vi "Colour detection subVI.vi"(2 "error in":errorcluster, 3 "Enum":T1(ring), 4 "Image In":T2) -> (0 "error out":errorcluster, 1 "Image overlay":T2(plugin-control))   [LabVIEW 2018]
uses:
  <vilib>/vision/Image Controls.llb/IMAQ Image.ctl
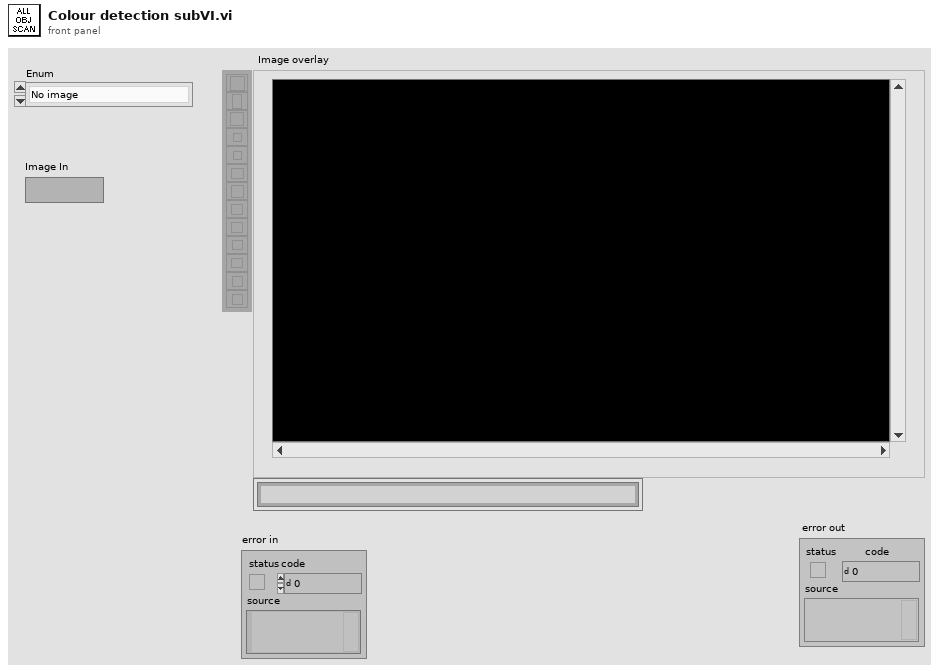
[diagram p1: front panel]
types:
  T1 = enum16{"No image", "Hair gel detection", "Pipe detection", "Ball detection", "Soap detection"}
  T2 = typedef "IMAQ Image.ctl" = refnum<image>
  T3 = cluster{"Desired Font (Application)":enum16{"User-specified Font", "Application Font", "System Font", "Dialog Font"}, "[User-specified Font]":cluster{"Font Name":string, "Size":i16, "Strikeout?":bool, "Italic?":bool, "Underline?":bool, "Outline?":bool, "Shadow?":bool, "Bold?":bool, "Rotation Angle":dbl}, "Horizontal Alignment":i16, "Vertical Alignment":i16}
  T4 = cluster{"Position":cluster{"x":sgl, "y":sgl}, "Angle":sgl, "Scale":sgl, "Score":sgl, "Bounding Box":cluster{"x":sgl, "y":sgl}[]}[]
  T5 = cluster{"Matches (Detect red)[0]":cluster{"Position":cluster{"x":sgl, "y":sgl}, "Angle":sgl, "Scale":sgl, "Score":sgl, "Bounding Box":cluster{"x":sgl, "y":sgl}[]}, "Matches (Detect red)[1]":cluster{"Position":cluster{"x":sgl, "y":sgl}, "Angle":sgl, "Scale":sgl, "Score":sgl, "Bounding Box":cluster{"x":sgl, "y":sgl}[]}, "Matches (Detect red)[2]":cluster{"Position":cluster{"x":sgl, "y":sgl}, "Angle":sgl, "Scale":sgl, "Score":sgl, "Bounding Box":cluster{"x":sgl, "y":sgl}[]}, "Matches (Detect red)[3]":cluster{"Position":cluster{"x":sgl, "y":sgl}, "Angle":sgl, "Scale":sgl, "Score":sgl, "Bounding Box":cluster{"x":sgl, "y":sgl}[]}, "Matches (Detect red)[4]":cluster{"Position":cluster{"x":sgl, "y":sgl}, "Angle":sgl, "Scale":sgl, "Score":sgl, "Bounding Box":cluster{"x":sgl, "y":sgl}[]}, "Matches (Detect red)[5]":cluster{"Position":cluster{"x":sgl, "y":sgl}, "Angle":sgl, "Scale":sgl, "Score":sgl, "Bounding Box":cluster{"x":sgl, "y":sgl}[]}, "Matches (Detect red)[6]":cluster{"Position":cluster{"x":sgl, "y":sgl}, "Angle":sgl, "Scale":sgl, "Score":sgl, "Bounding Box":cluster{"x":sgl, "y":sgl}[]}, "Matches (Detect red)[7]":cluster{"Position":cluster{"x":sgl, "y":sgl}, "Angle":sgl, "Scale":sgl, "Score":sgl, "Bounding Box":cluster{"x":sgl, "y":sgl}[]}, "Matches (Detect red)[8]":cluster{"Position":cluster{"x":sgl, "y":sgl}, "Angle":sgl, "Scale":sgl, "Score":sgl, "Bounding Box":cluster{"x":sgl, "y":sgl}[]}}
  T6 = cluster{"Bounding Box[0]":cluster{"x":sgl, "y":sgl}, "Bounding Box[1]":cluster{"x":sgl, "y":sgl}, "Bounding Box[2]":cluster{"x":sgl, "y":sgl}, "Bounding Box[3]":cluster{"x":sgl, "y":sgl}, "Bounding Box[4]":cluster{"x":sgl, "y":sgl}, "Bounding Box[5]":cluster{"x":sgl, "y":sgl}, "Bounding Box[6]":cluster{"x":sgl, "y":sgl}, "Bounding Box[7]":cluster{"x":sgl, "y":sgl}, "Bounding Box[8]":cluster{"x":sgl, "y":sgl}}
  T7 = cluster{"Global Rectangle":cluster{"x1Left":i32, "y1Top":i32, "x2Right":i32, "y2Bottom":i32}, "Centroid":cluster{"x":sgl, "y":sgl}, "Object Size":u32, "Score":dbl}[]
  T8 = cluster{"Shape Report (Shape Matching 1)[0]":cluster{"Global Rectangle":cluster{"x1Left":i32, "y1Top":i32, "x2Right":i32, "y2Bottom":i32}, "Centroid":cluster{"x":sgl, "y":sgl}, "Object Size":u32, "Score":dbl}, "Shape Report (Shape Matching 1)[1]":cluster{"Global Rectangle":cluster{"x1Left":i32, "y1Top":i32, "x2Right":i32, "y2Bottom":i32}, "Centroid":cluster{"x":sgl, "y":sgl}, "Object Size":u32, "Score":dbl}, "Shape Report (Shape Matching 1)[2]":cluster{"Global Rectangle":cluster{"x1Left":i32, "y1Top":i32, "x2Right":i32, "y2Bottom":i32}, "Centroid":cluster{"x":sgl, "y":sgl}, "Object Size":u32, "Score":dbl}, "Shape Report (Shape Matching 1)[3]":cluster{"Global Rectangle":cluster{"x1Left":i32, "y1Top":i32, "x2Right":i32, "y2Bottom":i32}, "Centroid":cluster{"x":sgl, "y":sgl}, "Object Size":u32, "Score":dbl}, "Shape Report (Shape Matching 1)[4]":cluster{"Global Rectangle":cluster{"x1Left":i32, "y1Top":i32, "x2Right":i32, "y2Bottom":i32}, "Centroid":cluster{"x":sgl, "y":sgl}, "Object Size":u32, "Score":dbl}, "Shape Report (Shape Matching 1)[5]":cluster{"Global Rectangle":cluster{"x1Left":i32, "y1Top":i32, "x2Right":i32, "y2Bottom":i32}, "Centroid":cluster{"x":sgl, "y":sgl}, "Object Size":u32, "Score":dbl}, "Shape Report (Shape Matching 1)[6]":cluster{"Global Rectangle":cluster{"x1Left":i32, "y1Top":i32, "x2Right":i32, "y2Bottom":i32}, "Centroid":cluster{"x":sgl, "y":sgl}, "Object Size":u32, "Score":dbl}, "Shape Report (Shape Matching 1)[7]":cluster{"Global Rectangle":cluster{"x1Left":i32, "y1Top":i32, "x2Right":i32, "y2Bottom":i32}, "Centroid":cluster{"x":sgl, "y":sgl}, "Object Size":u32, "Score":dbl}, "Shape Report (Shape Matching 1)[8]":cluster{"Global Rectangle":cluster{"x1Left":i32, "y1Top":i32, "x2Right":i32, "y2Bottom":i32}, "Centroid":cluster{"x":sgl, "y":sgl}, "Object Size":u32, "Score":dbl}}
  T9 = cluster{"Global Rectangle":cluster{"x1Left":i32, "y1Top":i32, "x2Right":i32, "y2Bottom":i32}, "Centroid":cluster{"x":sgl, "y":sgl}, "Object Size":u32, "Score":dbl}
  T10 = cluster{"x1Left":i32, "y1Top":i32, "x2Right":i32, "y2Bottom":i32}
  T11 = cluster{"Shape Report (calibrated) (Shape Matching 1)[0]":cluster{"Global Rectangle":cluster{"x1Left":i32, "y1Top":i32, "x2Right":i32, "y2Bottom":i32}, "Centroid":cluster{"x":sgl, "y":sgl}, "Object Size":u32, "Score":dbl}, "Shape Report (calibrated) (Shape Matching 1)[1]":cluster{"Global Rectangle":cluster{"x1Left":i32, "y1Top":i32, "x2Right":i32, "y2Bottom":i32}, "Centroid":cluster{"x":sgl, "y":sgl}, "Object Size":u32, "Score":dbl}, "Shape Report (calibrated) (Shape Matching 1)[2]":cluster{"Global Rectangle":cluster{"x1Left":i32, "y1Top":i32, "x2Right":i32, "y2Bottom":i32}, "Centroid":cluster{"x":sgl, "y":sgl}, "Object Size":u32, "Score":dbl}, "Shape Report (calibrated) (Shape Matching 1)[3]":cluster{"Global Rectangle":cluster{"x1Left":i32, "y1Top":i32, "x2Right":i32, "y2Bottom":i32}, "Centroid":cluster{"x":sgl, "y":sgl}, "Object Size":u32, "Score":dbl}, "Shape Report (calibrated) (Shape Matching 1)[4]":cluster{"Global Rectangle":cluster{"x1Left":i32, "y1Top":i32, "x2Right":i32, "y2Bottom":i32}, "Centroid":cluster{"x":sgl, "y":sgl}, "Object Size":u32, "Score":dbl}, "Shape Report (calibrated) (Shape Matching 1)[5]":cluster{"Global Rectangle":cluster{"x1Left":i32, "y1Top":i32, "x2Right":i32, "y2Bottom":i32}, "Centroid":cluster{"x":sgl, "y":sgl}, "Object Size":u32, "Score":dbl}, "Shape Report (calibrated) (Shape Matching 1)[6]":cluster{"Global Rectangle":cluster{"x1Left":i32, "y1Top":i32, "x2Right":i32, "y2Bottom":i32}, "Centroid":cluster{"x":sgl, "y":sgl}, "Object Size":u32, "Score":dbl}, "Shape Report (calibrated) (Shape Matching 1)[7]":cluster{"Global Rectangle":cluster{"x1Left":i32, "y1Top":i32, "x2Right":i32, "y2Bottom":i32}, "Centroid":cluster{"x":sgl, "y":sgl}, "Object Size":u32, "Score":dbl}, "Shape Report (calibrated) (Shape Matching 1)[8]":cluster{"Global Rectangle":cluster{"x1Left":i32, "y1Top":i32, "x2Right":i32, "y2Bottom":i32}, "Centroid":cluster{"x":sgl, "y":sgl}, "Object Size":u32, "Score":dbl}}
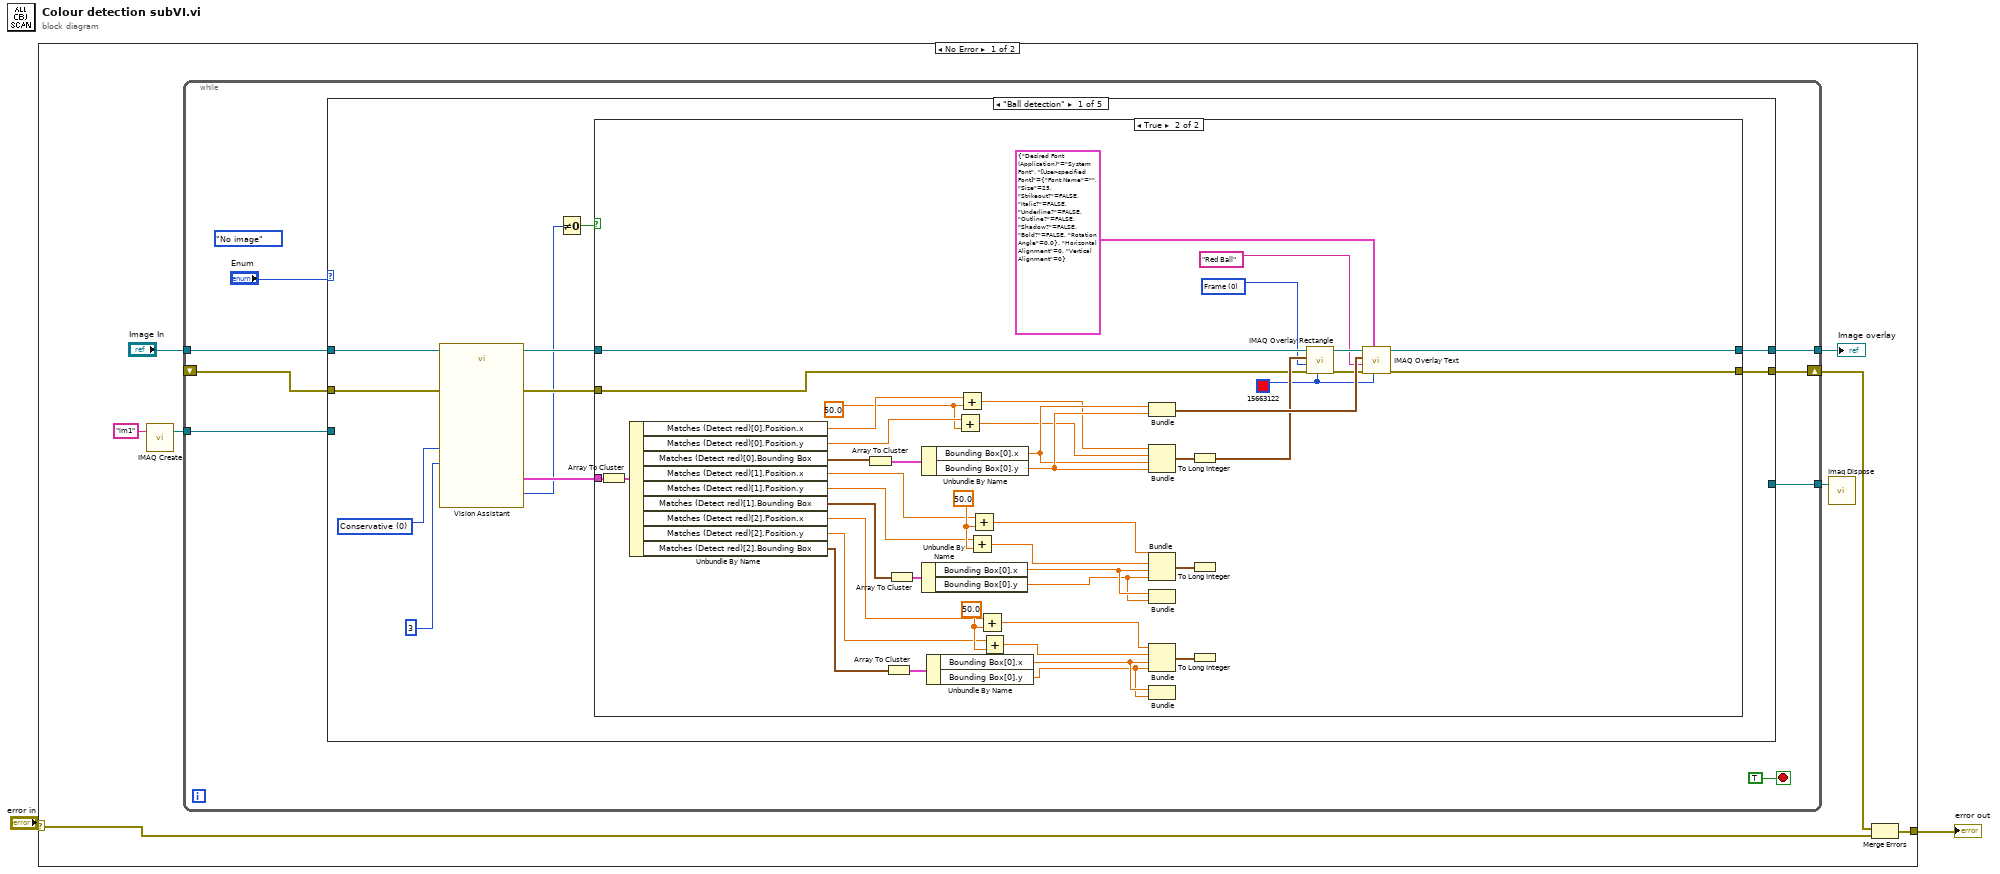
[diagram p0: block diagram]
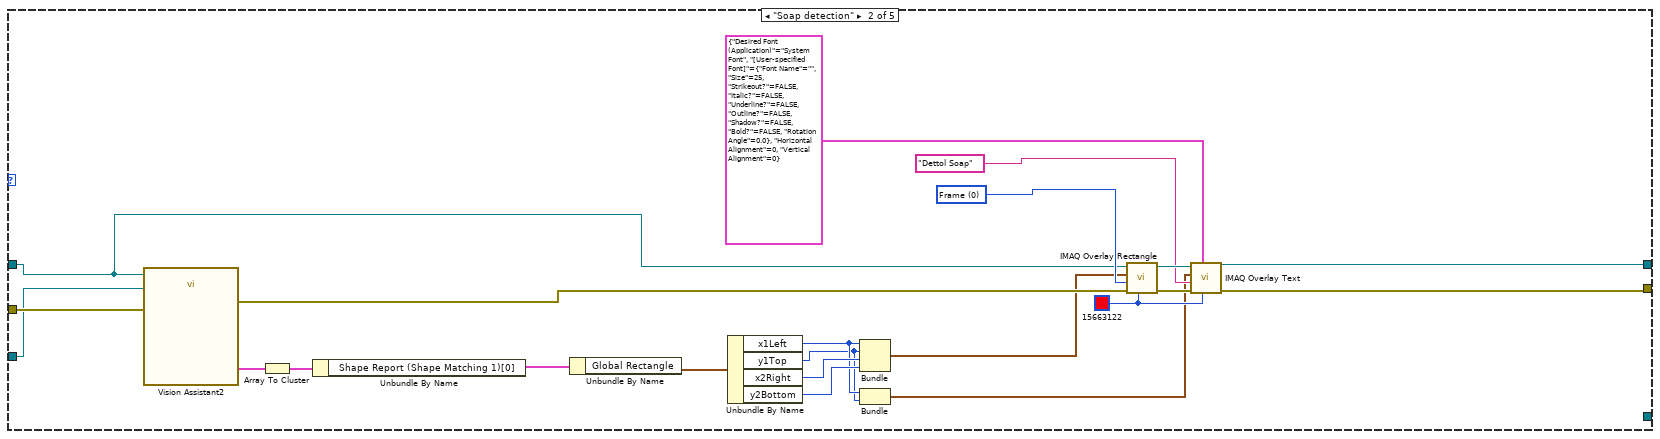
[diagram p3: hidden frame]
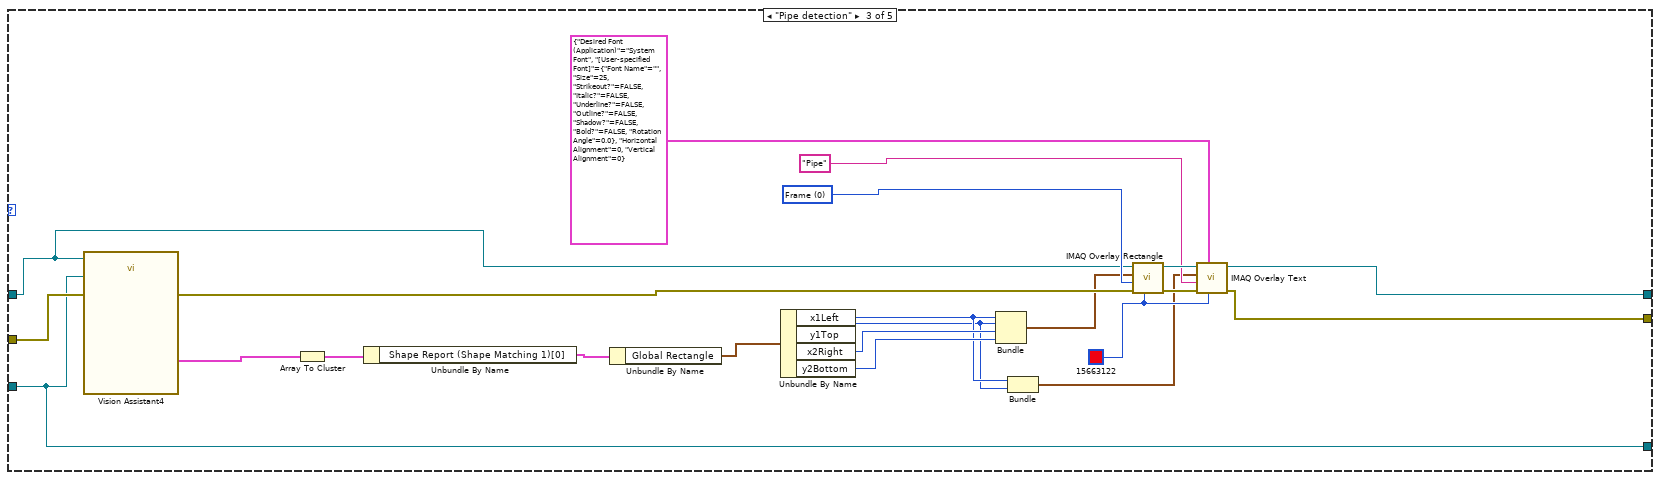
[diagram p4: hidden frame]
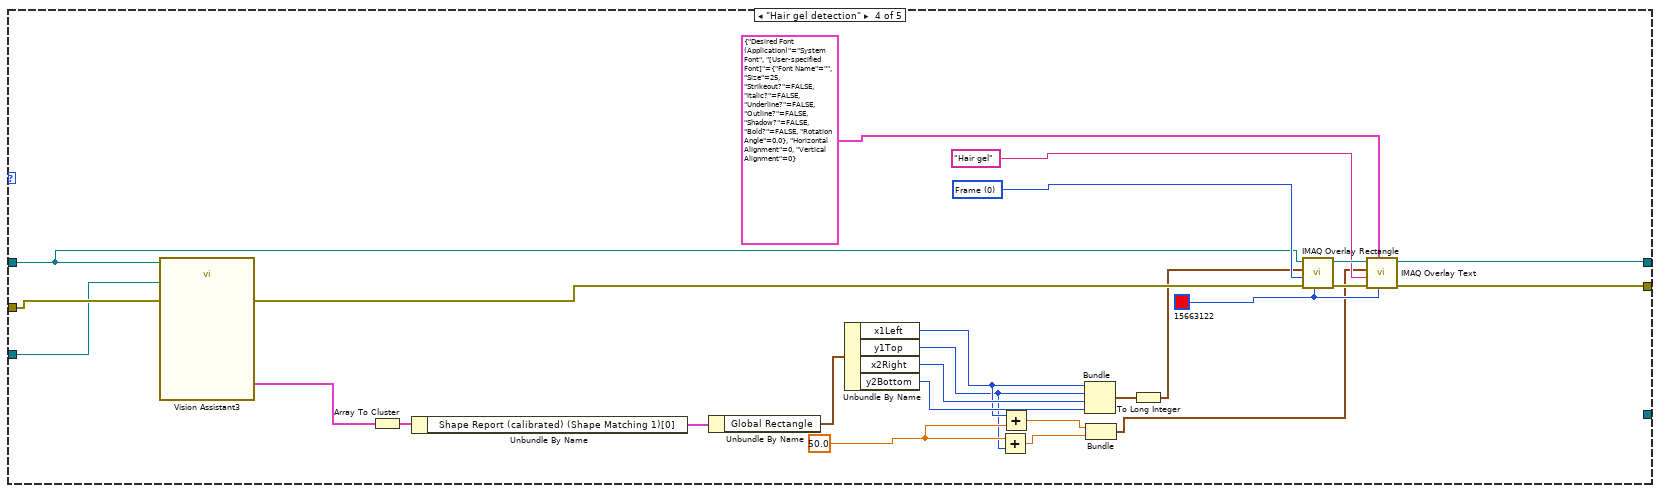
[diagram p5: hidden frame]
diagram:
  n1 = case shown="No Error" "error in" {
    selector: "error in" -> [w8 w148]
    tunnel: [w10 w148] -> w1
    frame No Error {
      n2 = call "IMAQ Create"("Image Name"="im1") -> ("New Image"=w4:T2)  [unwired: 4 in, 1 out]
      n3 = while {
        shift-right: [w17] -> w9
        shift-left: _ -> [w16]
        tunnel: "Image In" -> [w13]
        tunnel: [w14] -> w6
        tunnel: w4 -> [w12]
        tunnel: [w11] -> w3
        stop <- TRUE stop-if-true
        (unwired) T1."No image"
        n4 = case shown="\"Ball detection\"" "Enum" {
          tunnel: [w24 w78 w111 w135 w147] -> w17
          tunnel: w13 -> [w23 w76 w100 w121 _]
          tunnel: w16 -> [w22 w90 w119 w137 w147]
          tunnel: [w21 w79 w112 w136 _] -> w14
          tunnel: w12 -> [_ w77 w99 w120 w146]
          tunnel: [_ _ w99 _ w146] -> w11
          frame "Ball detection" {
            w27 = u32 0 items=["Conservative", "Balance", "Aggressive", "Very Aggressive"] ("Search Strategy (Detect red)")
            n5 = call "Vision Assistant"("Image In"=w23, "Search Strategy (Detect red)"=w27, "Number of Matches Requested (Detect red)"=3, "error in"=w22) -> ("Image Out"=w28:T2, "Matches (Detect red)"=w29:T4, "Number of Matches (Detect red)"=w19:i32, "error out"=w25:errorcluster)  [unwired: 20 in]
            n6 = Not Equal To 0?(x=w19) -> (x != 0?=w20:bool)
            n7 = case shown="True" w20 {
              tunnel: w29 -> [_ w75]
              tunnel: w28 -> [w31 w73]
              tunnel: w25 -> [w30 w35]
              tunnel: [w30 w32] -> w24
              tunnel: [w31 w33] -> w21
              frame False {
              }
              frame True {
                w46 = sgl 50.0 ("y")
                w57 = sgl 50.0 ("y")
                w58 = sgl 50.0 ("y")
                w34 = u32 15663122 ("Text Color (black)")
                w51 = u32 0 items=["Frame", "Fill", "Highlight"] ("Drawing Mode (Frame)")
                n8 = Array To Cluster(array=w75) -> (cluster=w74:T5)
                n9 = Unbundle By Name(w74) -> ("Matches (Detect red)[0].Position.x"=w64:sgl, "Matches (Detect red)[0].Position.y"=w62:sgl, "Matches (Detect red)[0].Bounding Box"=w72:cluster{"x":sgl, "y":sgl}[], "Matches (Detect red)[1].Position.x"=w56:sgl, "Matches (Detect red)[1].Position.y"=w55:sgl, "Matches (Detect red)[1].Bounding Box"=w60:cluster{"x":sgl, "y":sgl}[], "Matches (Detect red)[2].Position.x"=w45:sgl, "Matches (Detect red)[2].Position.y"=w44:sgl, "Matches (Detect red)[2].Bounding Box"=w47:cluster{"x":sgl, "y":sgl}[])
                n10 = Array To Cluster(array=w72) -> (cluster=w71:T6)
                n11 = Array To Cluster(array=w47) -> (cluster=w48:T6)
                n12 = Array To Cluster(array=w60) -> (cluster=w59:T6)
                n13 = Unbundle By Name(w59) -> ("Bounding Box[0].x"=w50:sgl, "Bounding Box[0].y"=w49:sgl)
                n14 = Unbundle By Name(w71) -> ("Bounding Box[0].x"=w65:sgl, "Bounding Box[0].y"=w68:sgl)
                n15 = Unbundle By Name(w48) -> ("Bounding Box[0].x"=w40:sgl, "Bounding Box[0].y"=w39:sgl)
                n16 = Add(x=w62, y=w58) -> (x+y=w61:sgl)
                n17 = Add(x=w64, y=w58) -> (x+y=w63:sgl)
                n18 = Add(x=w55, y=w57) -> (x+y=w53:sgl)
                n19 = Add(x=w56, y=w57) -> (x+y=w54:sgl)
                n20 = Add(x=w45, y=w46) -> (x+y=w43:sgl)
                n21 = Add(x=w44, y=w46) -> (x+y=w42:sgl)
                n22 = Bundle("x"=w65, "y"=w68) -> (w69:cluster{"x":sgl, "y":sgl})  [unwired: 1 in]
                n23 = Bundle(w63, w61, "x"=w65, "y"=w68) -> (w67:cluster{sgl, sgl, "x":sgl, "y":sgl})  [unwired: 1 in]
                n24 = Bundle(w54, w53, "x"=w50, "y"=w49) -> (w52:cluster{sgl, sgl, "x":sgl, "y":sgl})  [unwired: 1 in]
                n25 = Bundle("x"=w50, "y"=w49) -> ()  [unwired: 1 in, 1 out]
                n26 = Bundle(w43, w42, "x"=w40, "y"=w39) -> (w41:cluster{sgl, sgl, "x":sgl, "y":sgl})  [unwired: 1 in]
                n27 = Bundle("x"=w40, "y"=w39) -> ()  [unwired: 1 in, 1 out]
                n28 = To Long Integer(number=w67) -> (32bit integer=w66:cluster{i32, i32, "x":i32, "y":i32})
                n29 = To Long Integer(number=w52) -> ()  [unwired: 1 out]
                n30 = To Long Integer(number=w41) -> ()  [unwired: 1 out]
                n31 = call "IMAQ Overlay Rectangle"("Color"=w34, "error in (no error)"=w35, "Drawing Mode (Frame)"=w51, "Rectangle"=w66, "Image"=w73) -> ("error out"=w36:errorcluster, "Image Out"=w70:T2)  [unwired: 5 in]
                n32 = call "IMAQ Overlay Text"("Text Color (black)"=w34, "Font, Size & Style"=T3 {"Desired Font (Application)"=enum."System Font", "[User-specified Font]"={"Font Name"="", "Size"=25, "Strikeout?"=FALSE, "Italic?"=FALSE, "Underline?"=FALSE, "Outline?"=FALSE, "Shadow?"=FALSE, "Bold?"=FALSE, "Rotation Angle"=0.0}, "Horizontal Alignment"=0, "Vertical Alignment"=0}, "error in (no error)"=w36, "String"="Red Ball", "Origin"=w69, "Image"=w70) -> ("error out"=w32:errorcluster, "Image Out"=w33:T2)  [unwired: 4 in]
              }
            }
          }
          frame "Soap detection" {
            w91 = u32 15663122 ("Text Color (black)")
            w96 = u32 0 items=["Frame", "Fill", "Highlight"] ("Drawing Mode (Frame)")
            n33 = call "Vision Assistant2"("Image In"=w76, "Image Dst"=w77, "error in"=w90) -> ("Shape Report (Shape Matching 1)"=w89:T7, "error out"=w92:errorcluster)  [unwired: 21 in, 2 out]
            n34 = Array To Cluster(array=w89) -> (cluster=w88:T8)
            n35 = Unbundle By Name(w88) -> ("Shape Report (Shape Matching 1)[0]"=w87:T9)
            n36 = Unbundle By Name(w87) -> ("Global Rectangle"=w86:T10)
            n37 = Unbundle By Name(w86) -> ("x1Left"=w82:i32, "y1Top"=w81:i32, "x2Right"=w85:i32, "y2Bottom"=w84:i32)
            n38 = Bundle("x1Left"=w82, "y1Top"=w81, "x2Right"=w85, "y2Bottom"=w84) -> (w83:T10)  [unwired: 1 in]
            n39 = Bundle("x1Left"=w82, "y1Top"=w81) -> (w80:cluster{"x1Left":i32, "y1Top":i32})  [unwired: 1 in]
            n40 = call "IMAQ Overlay Rectangle"("Color"=w91, "error in (no error)"=w92, "Drawing Mode (Frame)"=w96, "Rectangle"=w83, "Image"=w76) -> ("error out"=w93:errorcluster, "Image Out"=w97:T2)  [unwired: 5 in]
            n41 = call "IMAQ Overlay Text"("Text Color (black)"=w91, "Font, Size & Style"=T3 {"Desired Font (Application)"=enum."System Font", "[User-specified Font]"={"Font Name"="", "Size"=25, "Strikeout?"=FALSE, "Italic?"=FALSE, "Underline?"=FALSE, "Outline?"=FALSE, "Shadow?"=FALSE, "Bold?"=FALSE, "Rotation Angle"=0.0}, "Horizontal Alignment"=0, "Vertical Alignment"=0}, "error in (no error)"=w93, "String"="Dettol Soap", "Origin"=w80, "Image"=w97) -> ("error out"=w78:errorcluster, "Image Out"=w79:T2)  [unwired: 4 in]
          }
          frame "Pipe detection" {
            w113 = u32 15663122 ("Text Color (black)")
            w117 = u32 0 items=["Frame", "Fill", "Highlight"] ("Drawing Mode (Frame)")
            n42 = call "Vision Assistant4"("Image In"=w100, "Image Dst"=w99, "error in"=w119) -> ("Shape Report (Shape Matching 1)"=w108:T7, "error out"=w110:errorcluster)  [unwired: 20 in, 3 out]
            n43 = Array To Cluster(array=w108) -> (cluster=w109:T8)
            n44 = Unbundle By Name(w109) -> ("Shape Report (Shape Matching 1)[0]"=w107:T9)
            n45 = Unbundle By Name(w107) -> ("Global Rectangle"=w106:T10)
            n46 = Unbundle By Name(w106) -> ("x1Left"=w103:i32, "y1Top"=w102:i32, "x2Right"=w105:i32, "y2Bottom"=w104:i32)
            n47 = Bundle("x1Left"=w103, "y1Top"=w102, "x2Right"=w105, "y2Bottom"=w104) -> (w98:T10)  [unwired: 1 in]
            n48 = Bundle("x1Left"=w103, "y1Top"=w102) -> (w101:cluster{"x1Left":i32, "y1Top":i32})  [unwired: 1 in]
            n49 = call "IMAQ Overlay Rectangle"("Color"=w113, "error in (no error)"=w110, "Drawing Mode (Frame)"=w117, "Rectangle"=w98, "Image"=w100) -> ("error out"=w114:errorcluster, "Image Out"=w118:T2)  [unwired: 5 in]
            n50 = call "IMAQ Overlay Text"("Text Color (black)"=w113, "Font, Size & Style"=T3 {"Desired Font (Application)"=enum."System Font", "[User-specified Font]"={"Font Name"="", "Size"=25, "Strikeout?"=FALSE, "Italic?"=FALSE, "Underline?"=FALSE, "Outline?"=FALSE, "Shadow?"=FALSE, "Bold?"=FALSE, "Rotation Angle"=0.0}, "Horizontal Alignment"=0, "Vertical Alignment"=0}, "error in (no error)"=w114, "String"="Pipe", "Origin"=w101, "Image"=w118) -> ("error out"=w111:errorcluster, "Image Out"=w112:T2)  [unwired: 4 in]
          }
          frame "Hair gel detection" {
            w138 = sgl 50.0 ("y")
            w139 = u32 15663122 ("Text Color (black)")
            w144 = u32 0 items=["Frame", "Fill", "Highlight"] ("Drawing Mode (Frame)")
            n51 = call "Vision Assistant3"("Image In"=w121, "Image Dst"=w120, "error in"=w137) -> ("Shape Report (calibrated) (Shape Matching 1)"=w123:T7, "error out"=w140:errorcluster)  [unwired: 20 in, 3 out]
            n52 = Array To Cluster(array=w123) -> (cluster=w134:T11)
            n53 = Unbundle By Name(w134) -> ("Shape Report (calibrated) (Shape Matching 1)[0]"=w122:T9)
            n54 = Unbundle By Name(w122) -> ("Global Rectangle"=w133:T10)
            n55 = Unbundle By Name(w133) -> ("x1Left"=w125:i32, "y1Top"=w124:i32, "x2Right"=w130:i32, "y2Bottom"=w129:i32)
            n56 = Add(x=w138, y=w124) -> (x+y=w131:sgl)
            n57 = Add(x=w125, y=w138) -> (x+y=w132:sgl)
            n58 = Bundle("x1Left"=w125, "y1Top"=w124, "x2Right"=w130, "y2Bottom"=w129) -> (w128:T10)  [unwired: 1 in]
            n59 = Bundle(w132, w131) -> (w126:cluster{sgl, sgl})  [unwired: 1 in]
            n60 = To Long Integer(number=w128) -> (32bit integer=w127:T10)
            n61 = call "IMAQ Overlay Rectangle"("Color"=w139, "error in (no error)"=w140, "Drawing Mode (Frame)"=w144, "Rectangle"=w127, "Image"=w121) -> ("error out"=w141:errorcluster, "Image Out"=w145:T2)  [unwired: 5 in]
            n62 = call "IMAQ Overlay Text"("Text Color (black)"=w139, "Font, Size & Style"=T3 {"Desired Font (Application)"=enum."System Font", "[User-specified Font]"={"Font Name"="", "Size"=25, "Strikeout?"=FALSE, "Italic?"=FALSE, "Underline?"=FALSE, "Outline?"=FALSE, "Shadow?"=FALSE, "Bold?"=FALSE, "Rotation Angle"=0.0}, "Horizontal Alignment"=0, "Vertical Alignment"=0}, "error in (no error)"=w141, "String"="Hair gel", "Origin"=w126, "Image"=w145) -> ("error out"=w135:errorcluster, "Image Out"=w136:T2)  [unwired: 4 in]
          }
          frame "No image", Default {
          }
        }
      }
      "Image overlay" <- w6
      n63 = call "Imaq Dispose"("Image"=w3) -> ()  [unwired: 5 in, 1 out]
      n64 = Merge Errors(w9, w8) -> (w10:errorcluster)
    }
    frame Error {
    }
  }
  "error out" <- w1
